vi "getWorkerList.vi"(8 "error in (no error)":errorcluster, 11 "BuildServer in":refnum<class "BuildServer.lvclass">) -> (0 "error out":errorcluster, 2 "Worker List":string[](array[string]), 3 "BuildServer out":refnum<class "BuildServer.lvclass">)   [LabVIEW 2017, in "BuildServer.lvlib" / "BuildServer.lvclass"]
uses:
  BuildServer.lvclass
  BuildServer.lvclass/BuildServer.ctl
  Classes/BuildWorker Interface/BuildWorker/BuildWorker.lvclass
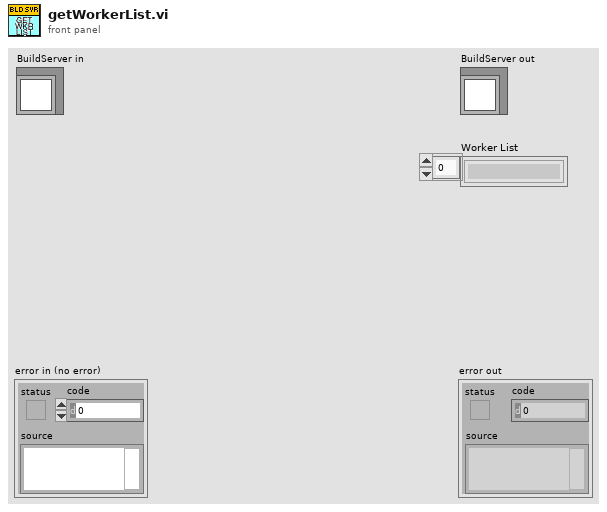
[diagram p1: front panel]
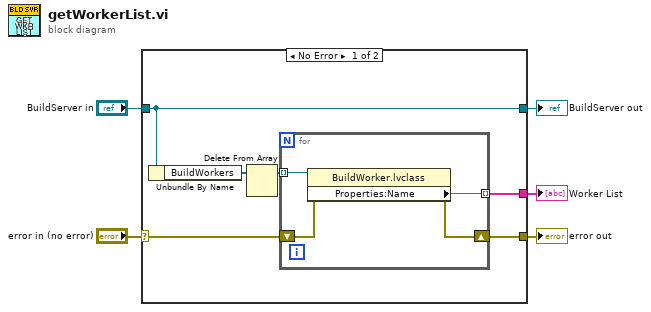
[diagram p0: block diagram]
diagram:
  n1 = case shown="No Error" "error in (no error)" {
    selector: "error in (no error)" -> [w10 w17]
    tunnel: [w9 w17] -> w4
    tunnel: [w11 w16] -> w2
    tunnel: "BuildServer in" -> [w11 w16]
    tunnel: [w8 _] -> w1
    frame No Error {
      n2 = Unbundle By Name(w11) -> ("BuildWorkers"=w7:refnum<class "BuildWorker.lvclass">[])
      n3 = Delete From Array(array=w7) -> (array with subset deleted=w6:refnum<class "BuildWorker.lvclass">[])  [unwired: 2 in, 1 out]
      n4 = for {
        tunnel: w6 -> [w15] mode=indexing
        tunnel: [w14] -> w8 mode=indexing
        shift-right: [w12] -> w9
        shift-left: w10 -> [w13]
        n5 = property class="BuildWorker.lvclass"(reference=w15, error in=w13) -> (error out=w12:errorcluster, "Properties:Name"=w14:string)  [unwired: 1 out]
      }
    }
    frame Error {
    }
  }
  "error out" <- w4
  "BuildServer out" <- w2
  "Worker List" <- w1
